vi "InitAppearance.vi"(8 "error in (no error)":errorcluster, 9 "Table Ref in":refnum<vi>, 10 "Col #":i32, 11 "DigitalCol in":refnum<class "DigitalCol.lvclass">) -> (0 "error out":errorcluster, 1 "Table Ref out":refnum<vi>, 3 "DigitalCol out":refnum<class "DigitalCol.lvclass">)   [LabVIEW 2013, in "DigitalCol.lvclass"]
doc: "Adds to Column:InitAppearance.vi (which sets column header, width, default colors) by coloring cells based on their value. No need to worry about disabled coloring here as it will be set later."
uses:
  DigitalCol.lvclass
  <vilib>/Utility/miscctls.llb/LVRowAndColumnTypeDef.ctl
  Column/Column.lvclass/Column.ctl
  Column/Column.lvclass
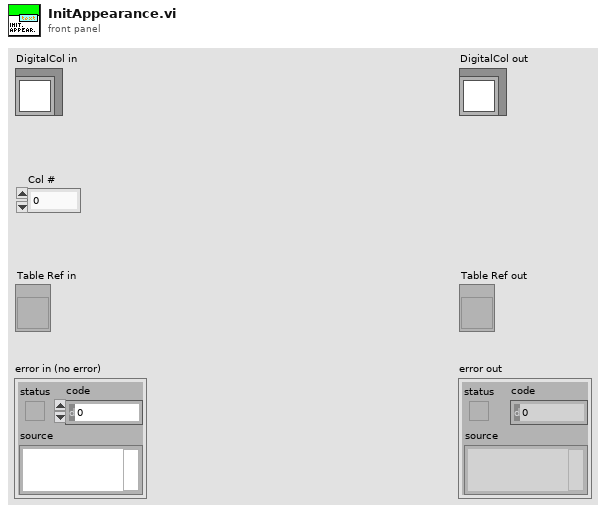
[diagram p1: front panel]
types:
  T1 = typedef "LVRowAndColumnTypeDef.ctl" = cluster{"Row":i32, "Column":i32}
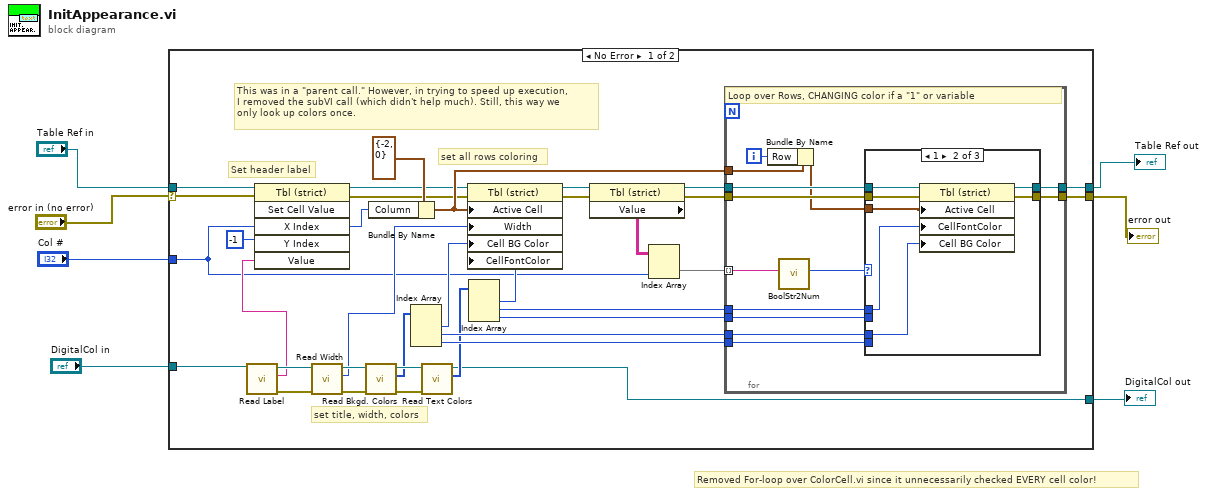
[diagram p0: block diagram]
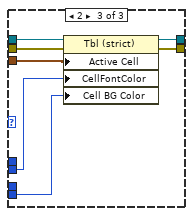
[diagram p3: hidden frame]
diagram:
  # "Removed For-loop over ColorCell.vi since it unnecessarily checked EVERY cell color!"
  n1 = case shown="No Error" "error in (no error)" {
    selector: "error in (no error)" -> [w8 w73]
    tunnel: [w14 w72] -> w3
    tunnel: [w13 w73] -> w4
    tunnel: "Table Ref in" -> [w12 w72]
    tunnel: "Col #" -> [w11 _]
    tunnel: "DigitalCol in" -> [w10 w71]
    tunnel: [w9 w71] -> w2
    frame No Error {
      # "This was in a \"parent call.\" However, in trying to speed up execution,\nI removed the subVI call (which didn't help much). Still, this way we\nonly look up colors once."
      # "Set header label"
      # "set title, width, colors"
      # "set all rows coloring"
      n2 = call "Read Label.vi"("Column in"=w10) -> ("error out"=w17:errorcluster, "Label"=w27:string, "Column out"=w30:refnum<class "DigitalCol.lvclass">)  [unwired: 8 in]
      n3 = invoke on="Invoke Node" class="Tbl (strict)" method="Set Cell Value"(reference=w12, error in=w8, "X Index"=w11, "Y Index"=-1 ("X Index"), "Value"=w27) -> (reference out=w19:refnum<vi>, error out=w18:errorcluster)  [unwired: 1 in, 4 out]
      n4 = call "Read Width.vi"("error in (no error)"=w17, "Column in"=w30) -> ("error out"=w16:errorcluster, "Width"=w20:u32, "Column out"=w29:refnum<class "DigitalCol.lvclass">)  [unwired: 7 in]
      n5 = call "Read Bkgd. Colors.vi"("error in (no error)"=w16, "Column in"=w29) -> ("error out"=w15:errorcluster, "Bkgd. Colors"=w22:u32[], "Column out"=w28:refnum<class "DigitalCol.lvclass">)  [unwired: 7 in]
      n6 = Bundle By Name(cluster=T1 {"Row"=-2, "Column"=0} ("RowAndCollumn"), "Column"=w11) -> (w41:T1)
      n7 = Index Array(array=w22) -> (element #1=w21:u32, element #2=w39:u32, element #3=w40:u32)  [unwired: 3 in]
      n8 = call "Read Text Colors.vi"("error in (no error)"=w15, "Column in"=w28) -> ("Text Colors"=w24:u32[], "Column out"=w9:refnum<class "DigitalCol.lvclass">)  [unwired: 7 in, 1 out]
      n9 = Index Array(array=w24) -> (element #1=w23:u32, element #2=w37:u32, element #3=w38:u32)  [unwired: 3 in]
      n10 = property class="Tbl (strict)"(reference=w19, error in=w18, "Active Cell"=w41, "Width"=w20, "Cell BG Color"=w21, "CellFontColor"=w23) -> (reference out=w32:refnum<vi>, error out=w33:errorcluster)
      n11 = property class="Tbl (strict)"(reference=w32, error in=w33) -> (reference out=w34:refnum<vi>, error out=w35:errorcluster, "Value"=w31:string[][])
      n12 = Index Array(array=w31, index (col)=w11) -> (element=w36:string[])  [unwired: 1 in]
      n13 = for {
        tunnel: w34 -> [w54]
        tunnel: w35 -> [w53]
        tunnel: w36 -> [w52] mode=indexing
        tunnel: w37 -> [w50]
        tunnel: w38 -> [w49]
        tunnel: w39 -> [w48]
        tunnel: w40 -> [w47]
        tunnel: w41 -> [w46]
        tunnel: [w43] -> w14
        tunnel: [w42] -> w13
        i -> [w45]
        # "Loop over Rows, CHANGING color if a \"1\" or variable"
        n14 = Bundle By Name(cluster=w46, "Row"=w45) -> (w44:T1)
        n15 = call "BoolStr2Num.vi"("Boolean string"=w52) -> ("number"=w51:i32)  [unwired: 10 in]
        n16 = case shown="1" w51 {
          tunnel: w54 -> [w56 w63 w70]
          tunnel: w53 -> [w55 w62 w69]
          tunnel: w50 -> [_ w61 _]
          tunnel: w49 -> [_ _ w68]
          tunnel: w48 -> [_ w60 _]
          tunnel: w47 -> [_ _ w67]
          tunnel: w44 -> [_ w59 w66]
          tunnel: [w56 w58 w65] -> w43
          tunnel: [w55 w57 w64] -> w42
          frame 0, Default {
            # "background/text colors\nalready set for \"0\"!"
          }
          frame 1 {
            n17 = property class="Tbl (strict)"(reference=w63, error in=w62, "Active Cell"=w59, "CellFontColor"=w61, "Cell BG Color"=w60) -> (reference out=w58:refnum<vi>, error out=w57:errorcluster)
          }
          frame 2 {
            n18 = property class="Tbl (strict)"(reference=w70, error in=w69, "Active Cell"=w66, "CellFontColor"=w68, "Cell BG Color"=w67) -> (reference out=w65:refnum<vi>, error out=w64:errorcluster)
          }
        }
      }
    }
    frame Error {
    }
  }
  "error out" <- w4
  "DigitalCol out" <- w2
  "Table Ref out" <- w3
